vi "Simulate Temperature Acquisition - Station 1.vi"() -> (3 "Temperature":dbl)   [LabVIEW 2019]
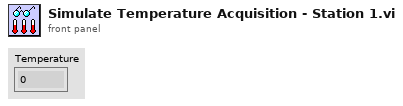
[diagram p1: front panel]
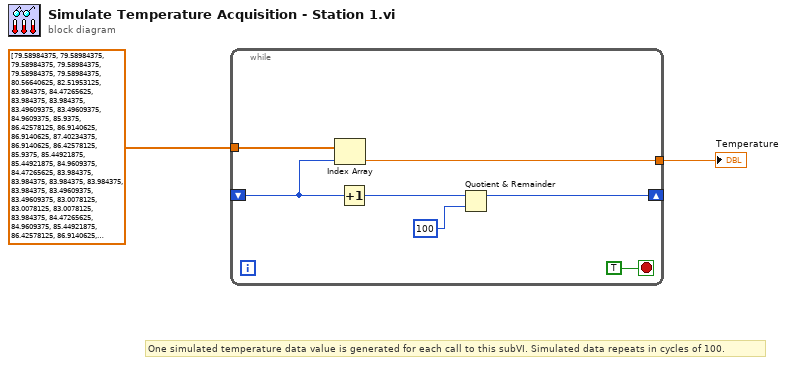
[diagram p0: block diagram]
diagram:
  # "One simulated temperature data value is generated for each call to this subVI. Simulated data repeats in cycles of 100."
  n1 = while {
    tunnel: dbl[] [79.58984375, 79.58984375, 79.58984375, 79.58984375, 79.58984375, 79.58984375, 80.56640625, 82.51953125, 83.984375, 84.47265625, 83.984375, 83.984375, 83.49609375, 83.49609375, 84.9609375, 85.9375, 86.42578125, 86.9140625, 86.9140625, 87.40234375, 86.9140625, 86.42578125, 85.9375, 85.44921875, 85.44921875, 84.9609375, 84.47265625, 83.984375, 83.984375, 83.984375, 83.984375, 83.984375, 83.49609375, 83.49609375, 83.0078125, 83.0078125, 83.0078125, 83.984375, 84.47265625, 84.9609375, 85.44921875, 86.42578125, 86.9140625, 86.9140625, 86.9140625, 86.42578125, 85.9375, 85.44921875, 85.9375, 86.9140625, 87.40234375, 87.890625, 87.40234375, 86.9140625, 86.9140625, 85.9375, 85.9375, 85.9375, 84.9609375, 84.9609375, 84.9609375, 84.47265625, 84.47265625, 85.44921875, 85.9375, 86.9140625, 86.9140625, 86.42578125, 85.9375, 85.44921875, 85.44921875, 84.9609375, 84.9609375, 84.47265625, 84.47265625, 83.984375, 83.984375, 83.49609375, 83.49609375, 83.0078125, 83.0078125, 83.0078125, 83.0078125, 83.0078125, 83.0078125, 83.0078125, 82.5193125, 81.0546875, 81.54296875, 82.5193125, 83.0078125, 82.51953125, 82.03125, 82.03125, 82.03125, 82.03125, 81.54296875, 81.54296875, 81.54296875, 81.54296875] ("array w/ subset deleted") -> [w8]
    tunnel: [w7] -> w2
    shift-right: [w5] -> _
    shift-left: _ -> [w3]
    stop <- TRUE stop-if-true
    n2 = Index Array(array=w8, index=w3) -> (element=w7:dbl)
    n3 = Increment(x=w3) -> (x+1=w4:i32)
    n4 = Quotient & Remainder(x=w4, y=100) -> (x-y*floor(x/y)=w5:i32)  [unwired: 1 out]
  }
  "Temperature" <- w2
